vi "DOE Configuration File Setup.vi"(8 "Error In":errorcluster) -> (0 "Error Out":errorcluster, 3 "Config File":string[][](array[string]))   [LabVIEW 2018]
panel:
  in  "Cycles Per Year":u32=5
  in  "Dryer PreCondition Enabled":string(combo)
  in  "Use Heise Barometric Pressure 901A":string(combo)
  in  "Standby Power Enabled":string(combo)
  in  "Reset Power Meter Enabled":string(combo)
  in  "Use Chroma?":string(combo)
  in  "Reset Hot Laurel Meter Enabled":string(combo)
  in  "Reset Cold Laurel Meter Enabled":string(combo)
  in  "Final RMC Enabled":string(combo)
  in  "Rinse Button Enabled":string(combo)
  in  "Dishwasher Events Visible":string(combo)
  in  "Boolean":bool
  in  "Max File Size":dbl=5.0
  in  "Station Name (Specific)":string
  in  "Agilent Gain":dbl=1.0
  in  "Cold Water Estimated Water Usage (Gallons)":dbl=20.0
  in  "Hot Water Estimated Water Usage (Gallons)":dbl=20.0
  in  "Time Limit At Power Level (Seconds)":dbl=3.0
  in  "Auto Terminate Power Limit (Watts)":dbl=2.0
  in  "Scan Rate":dbl=1.0
  in  "TC Type":string(combo)
  in  "Laurel Communication Type":string(combo)
  in  "Scale":string(combo)
  in  "Flow Rates":string(combo)
  in  "Analog DAQ":string(combo)
  in  "Power Analyzer":string(combo)
  in  "Test Stand Name":string(combo)
  out "Front Program Name":string="Parametric Stand"
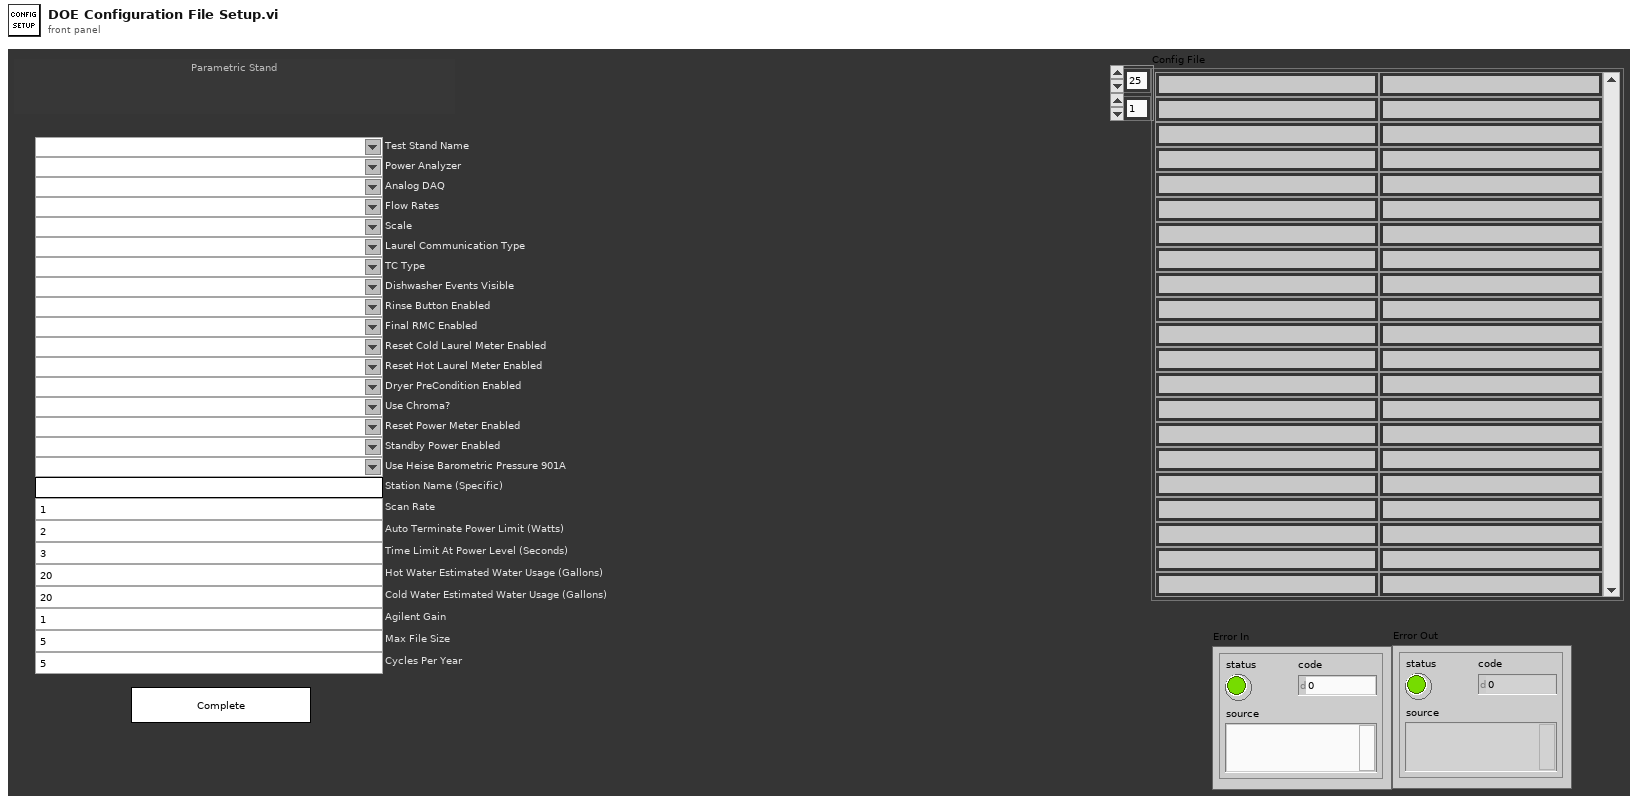
[diagram p1: front panel]
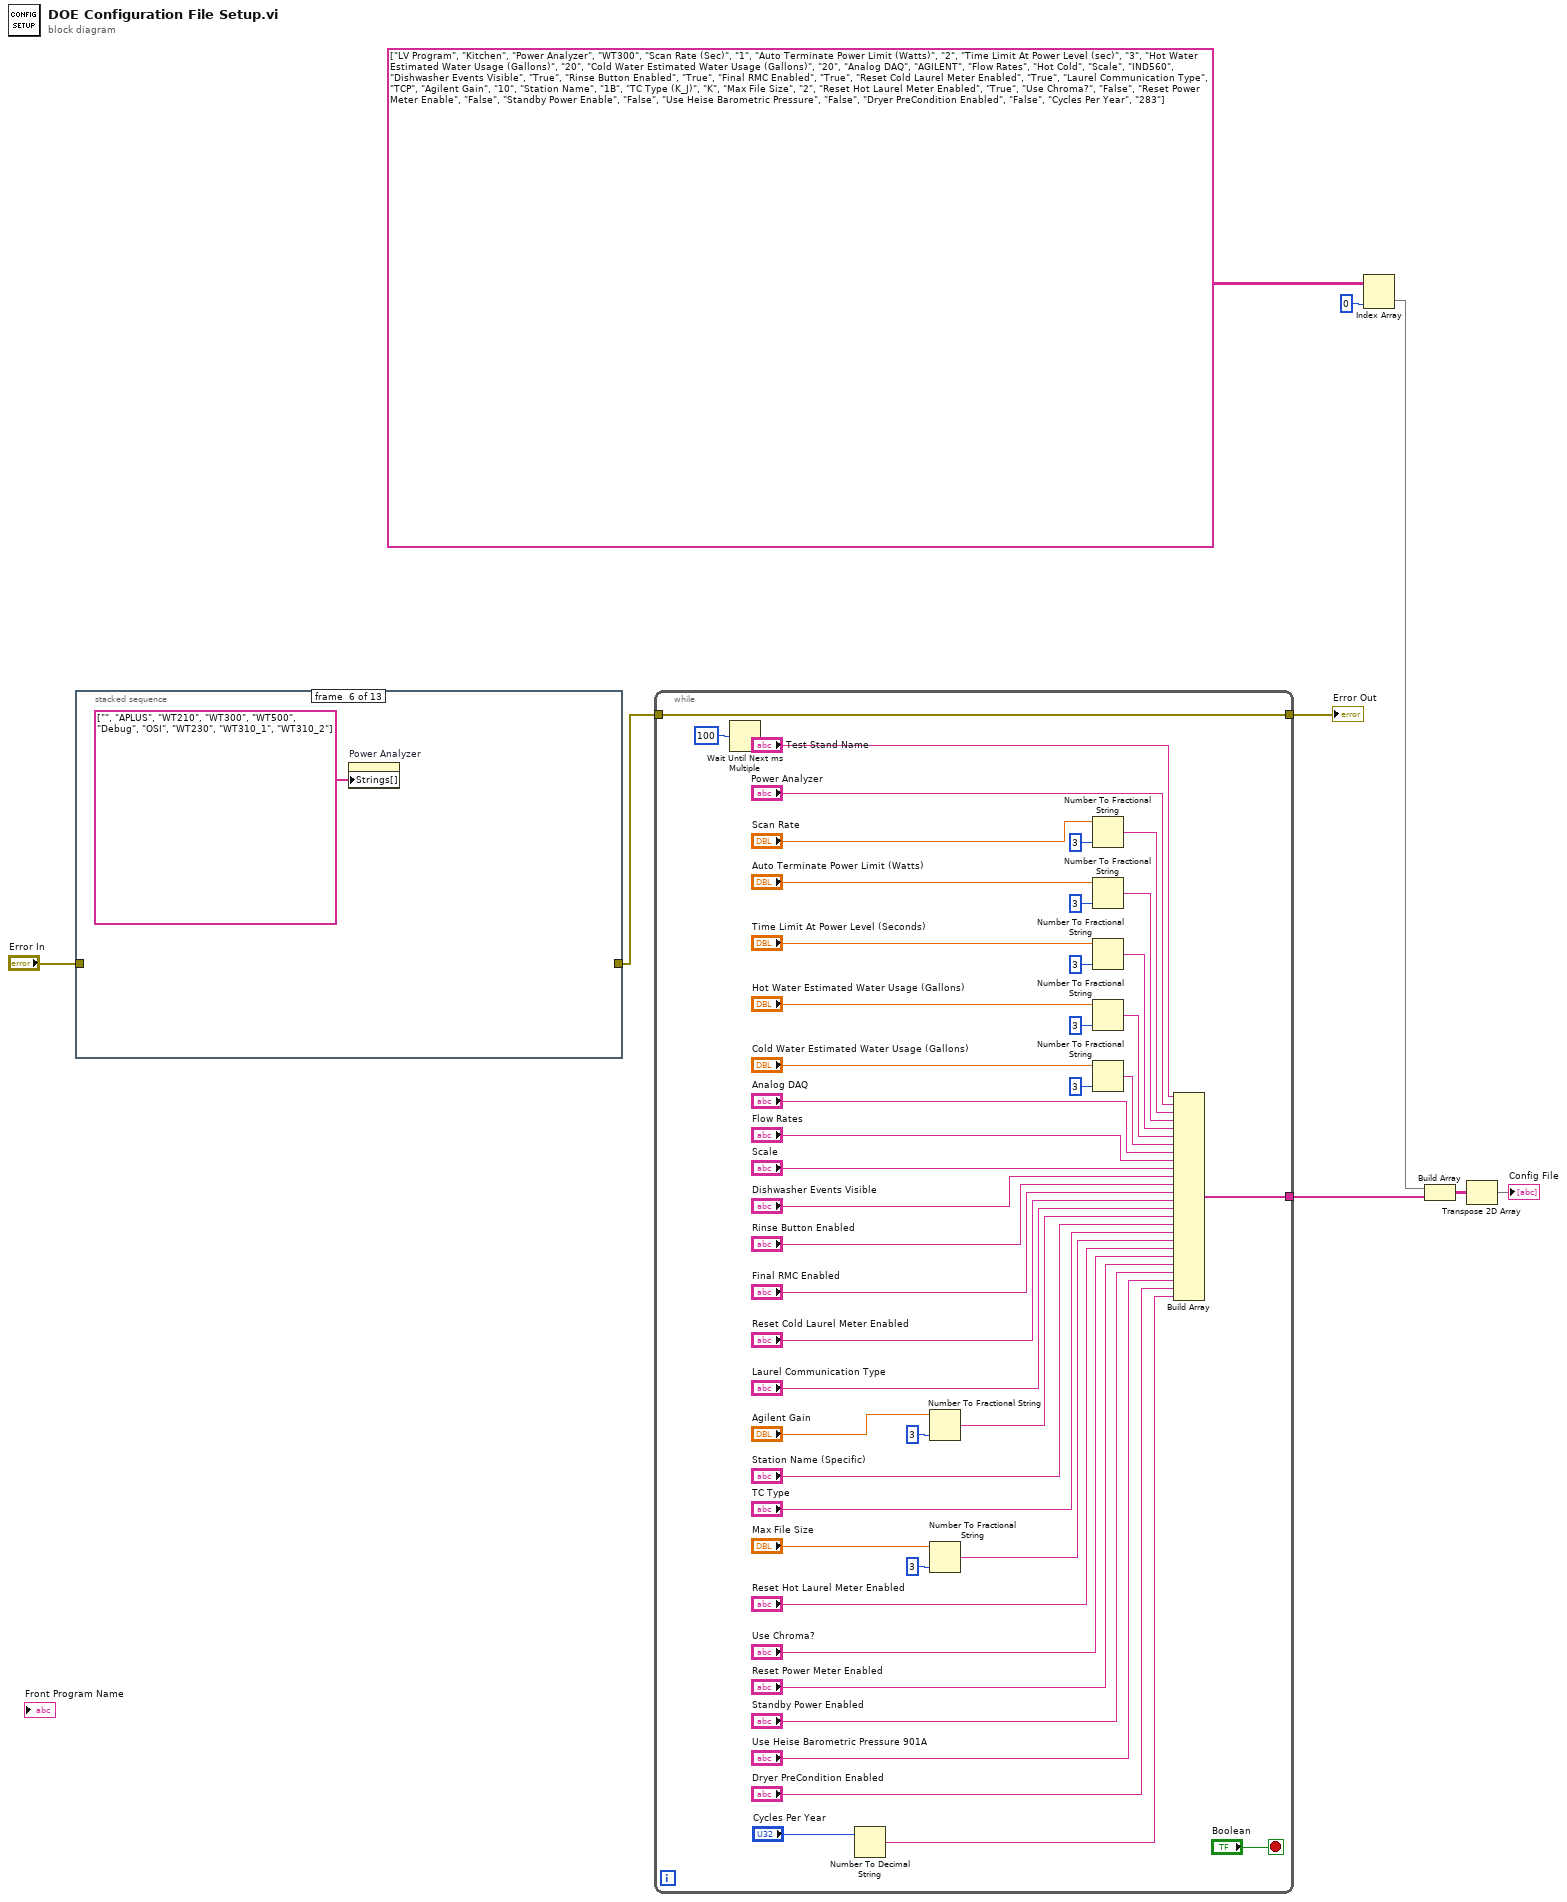
[diagram p0: block diagram]
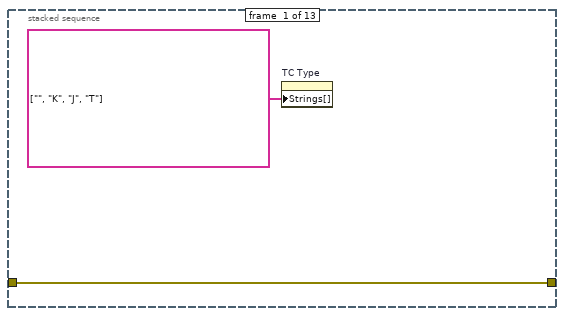
[diagram p2: hidden frame]
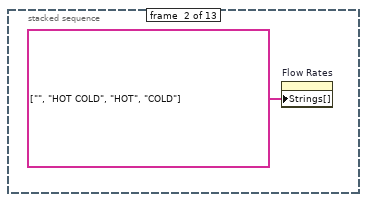
[diagram p3: hidden frame]
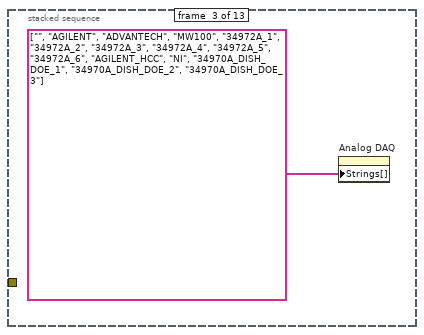
[diagram p4: hidden frame]
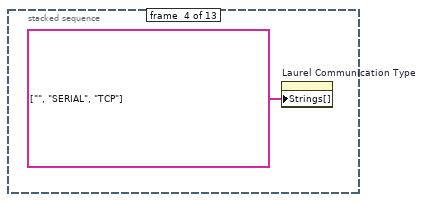
[diagram p5: hidden frame]
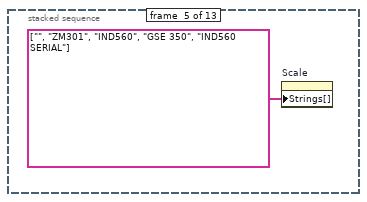
[diagram p6: hidden frame]
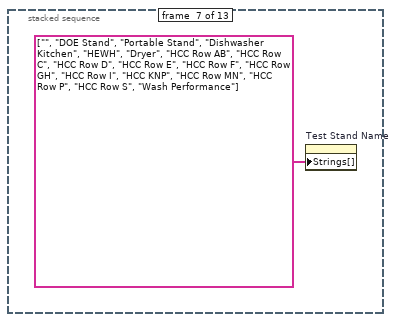
[diagram p7: hidden frame]
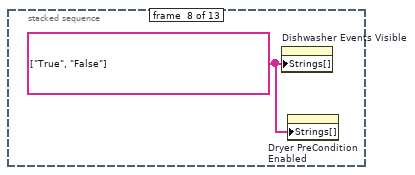
[diagram p8: hidden frame]
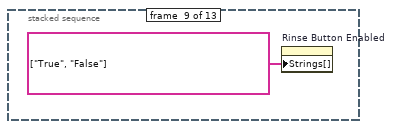
[diagram p9: hidden frame]
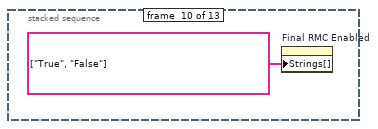
[diagram p10: hidden frame]
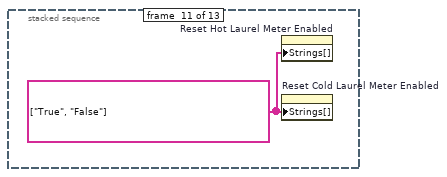
[diagram p11: hidden frame]
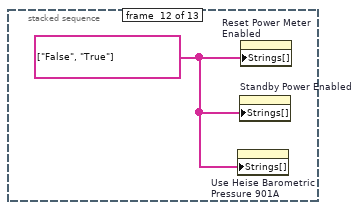
[diagram p12: hidden frame]
diagram:
  n1 = stacked-sequence {
    tunnel: "Error In" -> [w10 _ _ _ _ _ _ _ _ _ _ _ _]
    tunnel: [w10 _ _ _ _ _ _ _ _ _ _ _ _] -> w1
    frame #0 {
      n2 = property on="TC Type" class="CmbBox"("Strings[]"=string[] ["", "K", "J", "T"]) -> ()  [unwired: 2 in, 2 out]
    }
    frame #1 {
      n3 = property on="Flow Rates" class="CmbBox"("Strings[]"=string[] ["", "HOT COLD", "HOT", "COLD"]) -> ()  [unwired: 2 in, 2 out]
    }
    frame #2 {
      n4 = property on="Analog DAQ" class="CmbBox"("Strings[]"=string[] ["", "AGILENT", "ADVANTECH", "MW100", "34972A_1", "34972A_2", "34972A_3", "34972A_4", "34972A_5", "34972A_6", "AGILENT_HCC", "NI", "34970A_DISH_DOE_1", "34970A_DISH_DOE_2", "34970A_DISH_DOE_3"]) -> ()  [unwired: 2 in, 2 out]
    }
    frame #3 {
      n5 = property on="Laurel Communication Type" class="CmbBox"("Strings[]"=string[] ["", "SERIAL", "TCP"]) -> ()  [unwired: 2 in, 2 out]
    }
    frame #4 {
      n6 = property on="Scale" class="CmbBox"("Strings[]"=string[] ["", "ZM301", "IND560", "GSE 350", "IND560 SERIAL"]) -> ()  [unwired: 2 in, 2 out]
    }
    frame #5 {
      n7 = property on="Power Analyzer" class="CmbBox"("Strings[]"=string[] ["", "APLUS", "WT210", "WT300", "WT500", "Debug", "OSI", "WT230", "WT310_1", "WT310_2"]) -> ()  [unwired: 2 in, 2 out]
    }
    frame #6 {
      n8 = property on="Test Stand Name" class="CmbBox"("Strings[]"=string[] ["", "DOE Stand", "Portable Stand", "Dishwasher Kitchen", "HEWH", "Dryer", "HCC Row AB", "HCC Row C", "HCC Row D", "HCC Row E", "HCC Row F", "HCC Row GH", "HCC Row I", "HCC KNP", "HCC Row MN", "HCC Row P", "HCC Row S", "Wash Performance"]) -> ()  [unwired: 2 in, 2 out]
    }
    frame #7 {
      w18 = string[] ["True", "False"]
      n9 = property on="Dishwasher Events Visible" class="CmbBox"("Strings[]"=w18) -> ()  [unwired: 2 in, 2 out]
      n10 = property on="Dryer PreCondition Enabled" class="CmbBox"("Strings[]"=w18) -> ()  [unwired: 2 in, 2 out]
    }
    frame #8 {
      n11 = property on="Rinse Button Enabled" class="CmbBox"("Strings[]"=string[] ["True", "False"]) -> ()  [unwired: 2 in, 2 out]
    }
    frame #9 {
      n12 = property on="Final RMC Enabled" class="CmbBox"("Strings[]"=string[] ["True", "False"]) -> ()  [unwired: 2 in, 2 out]
    }
    frame #10 {
      w21 = string[] ["True", "False"]
      n13 = property on="Reset Hot Laurel Meter Enabled" class="CmbBox"("Strings[]"=w21) -> ()  [unwired: 2 in, 2 out]
      n14 = property on="Reset Cold Laurel Meter Enabled" class="CmbBox"("Strings[]"=w21) -> ()  [unwired: 2 in, 2 out]
    }
    frame #11 {
      w22 = string[] ["False", "True"] ("Strings []")
      n15 = property on="Use Heise Barometric Pressure 901A" class="CmbBox"("Strings[]"=w22) -> ()  [unwired: 2 in, 2 out]
      n16 = property on="Standby Power Enabled" class="CmbBox"("Strings[]"=w22) -> ()  [unwired: 2 in, 2 out]
      n17 = property on="Reset Power Meter Enabled" class="CmbBox"("Strings[]"=w22) -> ()  [unwired: 2 in, 2 out]
    }
    frame #12 {
    }
  }
  n18 = while {
    tunnel: w1 -> [w67]
    tunnel: [w67] -> w9
    tunnel: [w39] -> w5
    stop <- "Boolean" stop-if-true
    n19 = Wait Until Next ms Multiple(millisecond multiple=u32 100) -> ()  [unwired: 1 out]
    n20 = Number To Decimal String(number="Cycles Per Year") -> (decimal integer string=w23:string)  [unwired: 1 in]
    n21 = Number To Fractional String(number="Agilent Gain", precision (6)=i16 3) -> (F-format string=w43:string)  [unwired: 2 in]
    n22 = Number To Fractional String(number="Max File Size", precision (6)=i16 3) -> (F-format string=w40:string)  [unwired: 2 in]
    n23 = Number To Fractional String(number="Scan Rate", precision (6)=i16 3) -> (F-format string=w56:string)  [unwired: 2 in]
    n24 = Number To Fractional String(number="Auto Terminate Power Limit (Watts)", precision (6)=i16 3) -> (F-format string=w55:string)  [unwired: 2 in]
    n25 = Number To Fractional String(number="Time Limit At Power Level (Seconds)", precision (6)=i16 3) -> (F-format string=w54:string)  [unwired: 2 in]
    n26 = Number To Fractional String(number="Hot Water Estimated Water Usage (Gallons)", precision (6)=i16 3) -> (F-format string=w53:string)  [unwired: 2 in]
    n27 = Number To Fractional String(number="Cold Water Estimated Water Usage (Gallons)", precision (6)=i16 3) -> (F-format string=w52:string)  [unwired: 2 in]
    n28 = Build Array("Test Stand Name", "Power Analyzer", w56, w55, w54, w53, w52, "Analog DAQ", "Flow Rates", "Scale", "Dishwasher Events Visible", "Rinse Button Enabled", "Final RMC Enabled", "Reset Cold Laurel Meter Enabled", "Laurel Communication Type", w43, "Station Name (Specific)", "TC Type", w40, "Reset Hot Laurel Meter Enabled", "Use Chroma?", "Reset Power Meter Enabled", "Standby Power Enabled", "Use Heise Barometric Pressure 901A", "Dryer PreCondition Enabled", w23) -> (w39:string[])
  }
  "Error Out" <- w9
  n29 = Index Array(array=string[][] [["LV Program", "Kitchen"], ["Power Analyzer", "WT300"], ["Scan Rate (Sec)", "1"], ["Auto Terminate Power Limit (Watts)", "2"], ["Time Limit At Power Level (sec)", "3"], ["Hot Water Estimated Water Usage (Gallons)", "20"], ["Cold Water Estimated Water Usage (Gallons)", "20"], ["Analog DAQ", "AGILENT"], ["Flow Rates", "Hot Cold"], ["Scale", "IND560"], ["Dishwasher Events Visible", "True"], ["Rinse Button Enabled", "True"], ["Final RMC Enabled", "True"], ["Reset Cold Laurel Meter Enabled", "True"], ["Laurel Communication Type", "TCP"], ["Agilent Gain", "10"], ["Station Name", "1B"], ["TC Type (K_J)", "K"], ["Max File Size", "2"], ["Reset Hot Laurel Meter Enabled", "True"], ["Use Chroma?", "False"], ["Reset Power Meter Enable", "False"], ["Standby Power Enable", "False"], ["Use Heise Barometric Pressure", "False"], ["Dryer PreCondition Enabled", "False"], ["Cycles Per Year", "283"]], index (col)=0 ("disabled index (col)")) -> (element=w6:string[])  [unwired: 1 in]
  n30 = Build Array(w6, w5) -> (w4:string[][])
  n31 = Transpose 2D Array(2D array=w4) -> (transposed array=→"Config File":string[][])
